vi "Get Listbox Item.vi"(8 "error in (no error)":errorcluster) -> (0 "error out":errorcluster, 2 "OK?":bool, 3 "Item out":string)   [LabVIEW 2020, in "Instrument Addon System Explorer.lvlib"]
uses:
  Instrument Addon System Explorer.lvlib
panel:
  in  "Cancel":bool
  in  "OK":bool
  in  "New Item":string
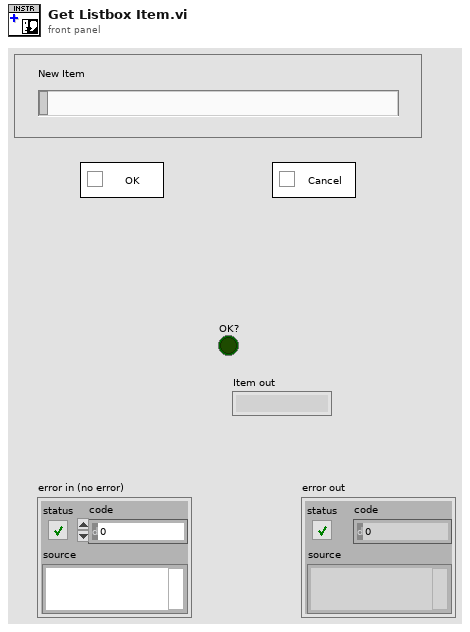
[diagram p1: front panel]
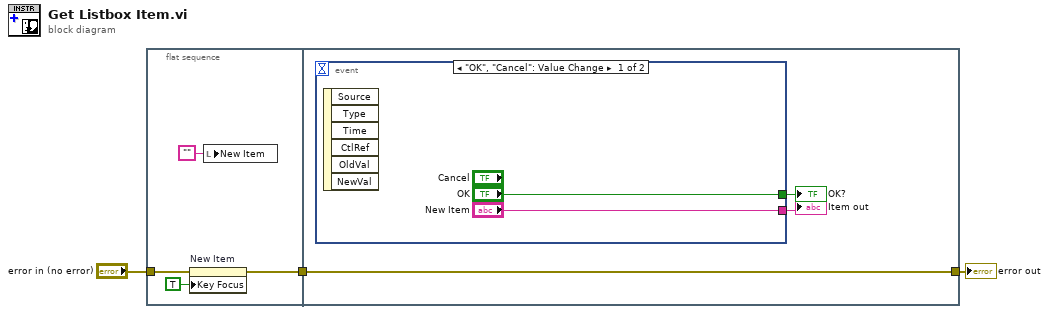
[diagram p0: block diagram]
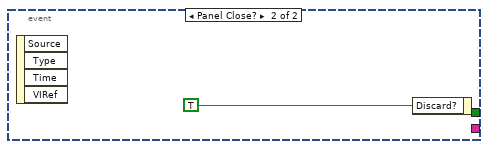
[diagram p2: hidden frame]
diagram:
  n1 = flat-sequence {
    tunnel: [w5] -> w2
    tunnel: "error in (no error)" -> [w6]
    tunnel: [w8] -> w3
    tunnel: w2 -> [w8]
    frame #0 {
      n2 = property on="New Item" class="Str"(error in=w6, "Key Focus"=TRUE) -> (error out=w5:errorcluster)  [unwired: 1 in, 1 out]
      n3 = local write "New Item"("") -> ()
    }
    frame #1 {
      n4 = event shown="[0] \"OK\", \"Cancel\": Value Change" {
        selector: _ -> [_ _]
        dyn-events: _ -> [_ _]
        timeout: _ -> [_ _]
        tunnel: ["OK" _] -> w10
        tunnel: ["New Item" _] -> w9
        event "OK", "Cancel": Value Change {
          n5 = event-data() -> ()  [unwired: 1 in, 6 out]
        }
        event Panel Close? {
          n6 = event-data() -> ()  [unwired: 1 in, 4 out]
          n7 = event-data("Discard?"=TRUE) -> ()  [unwired: 1 in, 1 out]
        }
      }
      "OK?" <- w10
      "Item out" <- w9
    }
  }
  "error out" <- w3
